vi "TDC_getVersion.vi"() -> (3 "Library Version":dbl)   [LabVIEW 2011]
uses:
  tdcbase.dll
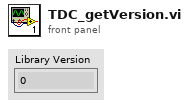
[diagram p1: front panel]
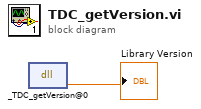
[diagram p0: block diagram]
diagram:
  n1 = dll-call lib="X:/tdcbase.dll" fn="_TDC_getVersion@0"() -> ("return type"=→"Library Version":dbl)  [unwired: 3 in, 2 out]
